vi "Image Processing Handler Initialize Events.vi"(8 "error in (no error)":errorcluster, 11 "Image Processing Handler in":refnum<class "Image Processing Handler.lvclass">) -> (0 "error out":errorcluster, 2 "Event Registration Refnum":refnum<event-registration>, 3 "Image Processing Handler out":refnum<class "Image Processing Handler.lvclass">)   [LabVIEW 2018, in "Image Processing Handler.lvclass"]
uses:
  Image Processing Handler.lvclass
  Message/Message.lvclass
  Image Processing Handler.lvclass/Image Processing Handler.ctl
  Image Processing Module Event Handler.vi
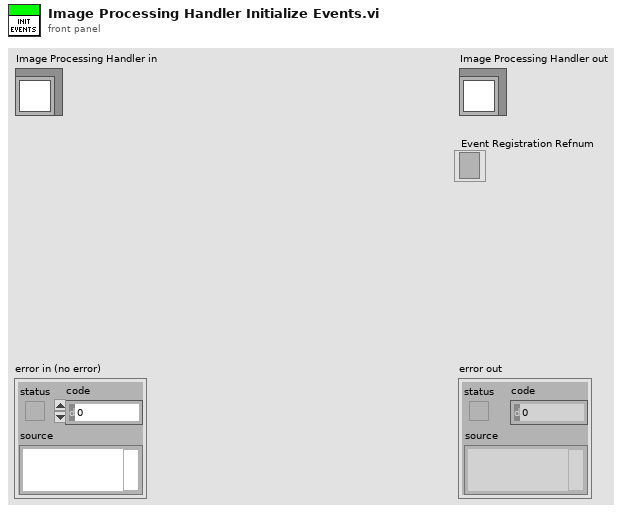
[diagram p1: front panel]
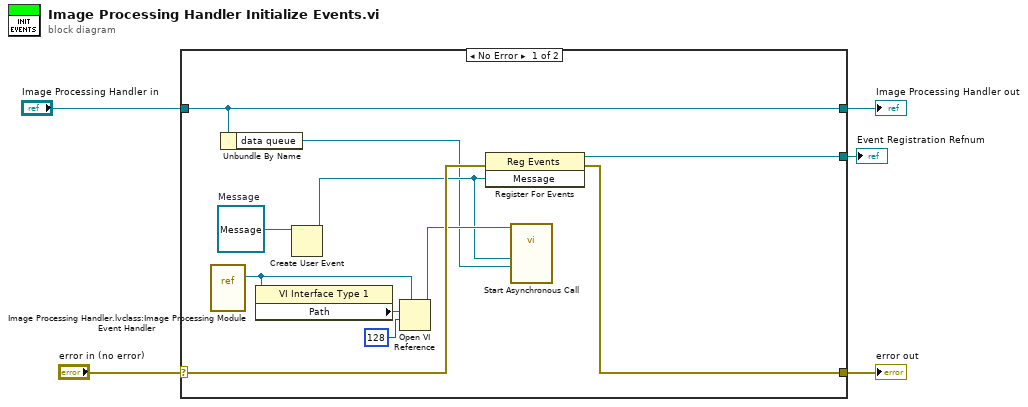
[diagram p0: block diagram]
diagram:
  n1 = case shown="No Error" "error in (no error)" {
    selector: "error in (no error)" -> [w16 w18]
    tunnel: [w15 w18] -> w4
    tunnel: [w7 w17] -> w2
    tunnel: "Image Processing Handler in" -> [w7 w17]
    tunnel: [w14 _] -> w1
    frame No Error {
      w13 = refnum<class "Message.lvclass"> refnum  # Message
      n2 = vi-ref "Image Processing Handler.lvclass:Image Processing Module Event Handler.vi"() -> (w9:refnum<vi>)
      n3 = Unbundle By Name(w7) -> ("data queue"=w6:refnum<queue>)
      n4 = property class="VI Interface Type 1"(reference=w9) -> ("Path"=w12:path)  [unwired: 1 in, 2 out]
      n5 = Create User Event(user event datatype=w13) -> (user event=w8:refnum<user-event>)  [unwired: 1 in, 1 out]
      n6 = Open VI Reference(type specifier VI Refnum (for type only)=w9, vi path=w12, options=128) -> (vi reference=w10:refnum<vi>)  [unwired: 3 in, 1 out]
      n7 = register-events(error in=w16, w8) -> (reference out=w14:refnum<event-registration>, error out=w15:errorcluster)  [unwired: 1 in]
      n8 = call-by-ref "Start Asynchronous Call"(reference=w10, "data queue"=w6, "Data Event"=w8) -> ()  [unwired: 11 in, 2 out]
    }
    frame Error {
    }
  }
  "error out" <- w4
  "Image Processing Handler out" <- w2
  "Event Registration Refnum" <- w1
